vi "Variant_ExtractClusterElementByName.vi"(9 "name":string, 11 "Cluster":variant) -> (1 "index":i32=-1, 2 "Element":variant, 3 "Cluster dup":variant)   [LabVIEW 2013, in "OpenVariant.lvlib"]
uses:
  OpenVariant.lvlib
  TypeDescriptor/OpenDescriptor.lvlib
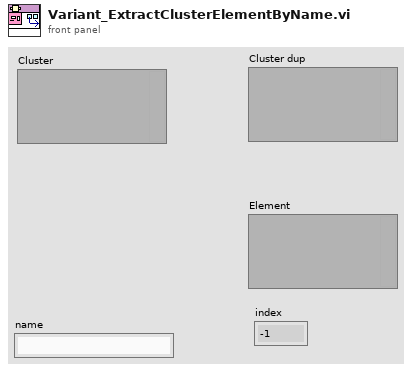
[diagram p1: front panel]
types:
  T1 = typedef "OpenDescriptor.lvlib/OpenDescriptor -- cluster.ctl" = cluster{"type descriptor":i16[], "name":string, "class":string, "data string":string}
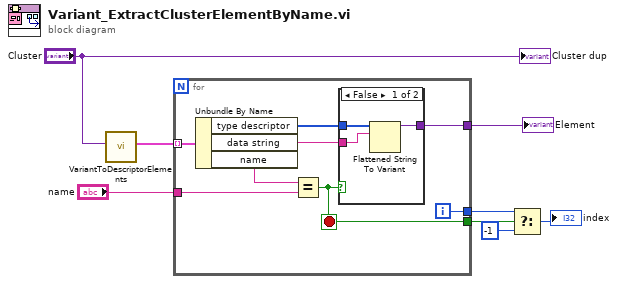
[diagram p0: block diagram]
diagram:
  n1 = call "VariantToDescriptorElements.vi"("Variant"="Cluster") -> ("Descriptors"=w1:T1[])  [unwired: 9 in, 1 out]
  n2 = for {
    tunnel: w1 -> [w16] mode=indexing
    tunnel: "name" -> [w14]
    tunnel: [w11] -> w7
    tunnel: [w10] -> w6
    tunnel: [w9] -> w5
    i -> [w9]
    stop <- w10 stop-if-true
    n3 = Unbundle By Name(w16) -> ("type descriptor"=w13:i16[], "data string"=w12:string, "name"=w15:string)
    n4 = Equal?(x=w15, y=w14) -> (x = y?=w10:bool)
    n5 = case shown="False" w10 {
      tunnel: w13 -> [w19 _]
      tunnel: w12 -> [w18 _]
      tunnel: [w17 _] -> w11
      frame False {
        n6 = Flattened String To Variant(6:w18, 7:w19) -> (3:w17:variant)  [unwired: 1 in, 1 out]
      }
      frame True {
      }
    }
  }
  "Element" <- w7
  n7 = Select(t=w5, s=w6, f=-1) -> (s? t:f=→"index":i32)
  "Cluster dup" <- "Cluster"
